vi "Curvature of Bezier Curve.vi"(10 "percision":dbl, 11 "ctrl points":cluster{dbl, dbl}[](array[cluster])) -> (3 "curvature":dbl[](array[numeric]))   [LabVIEW 2019]
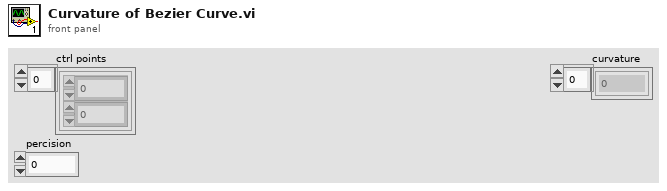
[diagram p1: front panel]
types:
  T1 = typedef "Bezier Curve.ctl" = cluster{"x":dbl, "y":dbl}[]
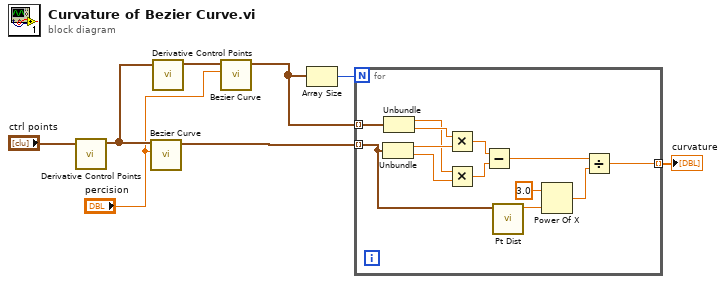
[diagram p0: block diagram]
diagram:
  n1 = call "Derivative Control Points.vi"("ctrl points"="ctrl points") -> ("d ctrl pts"=w7:cluster{dbl, dbl}[])  [unwired: 10 in]
  n2 = call "Bezier Curve.vi"("percision"="percision", "ctrl points"=w7) -> ("curve"=w2:T1)  [unwired: 9 in]
  n3 = call "Derivative Control Points.vi"("ctrl points"=w7) -> ("d ctrl pts"=w6:cluster{dbl, dbl}[])  [unwired: 10 in]
  n4 = call "Bezier Curve.vi"("percision"="percision", "ctrl points"=w6) -> ("curve"=w3:T1)  [unwired: 9 in]
  n5 = Array Size(array=w3) -> (size(s)=w4:i32)
  n6 = for {
    N: w4 -> [_]
    tunnel: w3 -> [w21] mode=indexing
    tunnel: w2 -> [w13] mode=indexing
    tunnel: [w9] -> w1 mode=indexing
    n7 = Unbundle(w13) -> ("x"=w20:dbl, "y"=w17:dbl)
    n8 = Unbundle(w21) -> ("x"=w18:dbl, "y"=w19:dbl)
    n9 = Multiply(x=w19, y=w20) -> (x*y=w15:dbl)
    n10 = Multiply(x=w18, y=w17) -> (x*y=w16:dbl)
    n11 = Subtract(x=w15, y=w16) -> (x-y=w14:dbl)
    n12 = call "Pt Dist.vi"("point a"=w13) -> ("dist"=w12:dbl)  [unwired: 10 in]
    n13 = Power Of X(1:w12, 2:3.0 ("y")) -> (0:w10:dbl)
    n14 = Divide(x=w14, y=w10) -> (x/y=w9:dbl)
  }
  "curvature" <- w1
